vi "Periodic Tasks - working_old.vi"(8 "error in":errorcluster) -> ()   [LabVIEW 2017]
doc: "This VI runs in parallel to other tasks. It can contain as many user-defined periodic loops as you need. These can carry out PID or other sorts of timed response."
uses:
  <vilib>/Analysis/baseanly.llb/Mean (DBL).vi
  <vilib>/Rock Robotics/WPI/Utilities/WPI_GetSetVariantRefNum.vi
  Robot Global Data.vi
  <vilib>/Analysis/NI_AALBase.lvlib
panel:
  out "Avg Y":dbl
  out "Mean":dbl(graph)
  out "Joy Y":dbl(graph)
  out "Current Joy Y Value":dbl
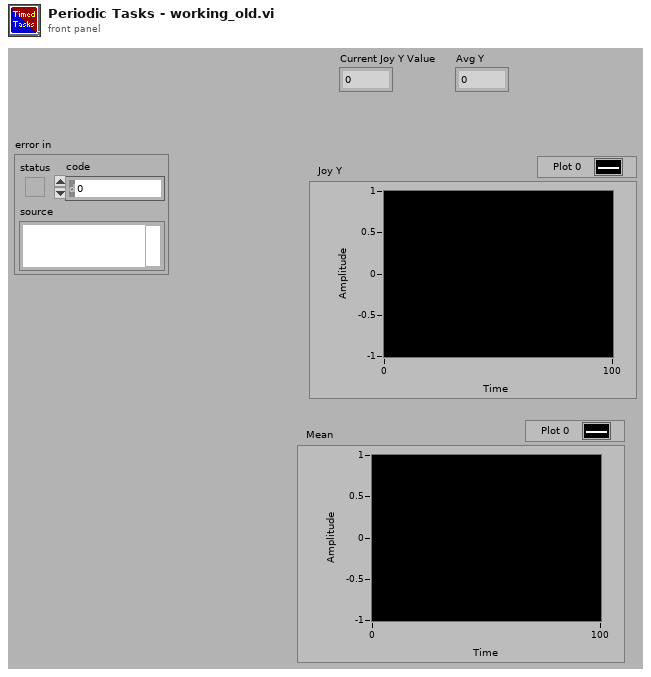
[diagram p1: front panel]
types:
  T1 = typedef "WPI_JoystickDevRef.ctl" = cluster{"Device":T2}
  T2 = typedef "WPI_JoystickDeviceEnum.ctl" = enum16{"USB 0", "USB 1", "USB 2", "USB 3", "USB 4", "USB 5"}
  T3 = typedef "WPI_RobotDriveDevRef.ctl" = cluster{"DevStatus":errorcluster, "Motors[]":T4[], "Square Inputs":bool, "Max Output":dbl}
  T4 = typedef "WPI_MotorControlDeviceRef.ctl" = cluster{"DeviceStatus":errorcluster, "Type":T5, "PWM":cluster{"PWM Channel":T6, "DeadBand":T7}, "CAN":cluster{"Device Number":u8, "SetOutput VI Ref":variant, "GetOutput VI Ref":variant, "Enable VI Ref":variant, "Disable VI Ref":variant, "Data":variant}, "Invert":bool, "DIO PWM":cluster{"PWM \"Enable\" Channel":T6, "DIOChannel":T8, "PWM Rate":dbl}}
  T5 = typedef "WPI_MotorControlType.ctl" = enum16{"PWM", "CAN", "DIO PWM"}
  T6 = typedef "FPGA_DIOPWMChannel.ctl" = enum8{"PWM 0", "PWM 1", "PWM 2", "PWM 3", "PWM 4", "PWM 5", "PWM 6", "PWM 7", "PWM 8", "PWM 9", "PWM MXP 0", "PWM MXP 1", "PWM MXP 2", "PWM MXP 3", "PWM MXP 4", "PWM MXP 5", "PWM MXP 6", "PWM MXP 7", "PWM MXP 8", "PWM MXP 9", "Invalid"}
  T7 = typedef "WPI_PWMDeadband.ctl" = cluster{"Name":string, "maxPositivePwm":i32, "minPositivePwm":i32, "centerPwm":i32, "maxNegativePwm":i32, "minNegativePwm":i32, "angularRange":u16}
  T8 = typedef "FPGA_DIOChannel.ctl" = enum8{"DIO 0", "DIO 1", "DIO 2", "DIO 3", "DIO 4", "DIO 5", "DIO 6", "DIO 7", "DIO 8", "DIO 9", "DIO MXP 0", "DIO MXP 1", "DIO MXP 2", "DIO MXP 3", "DIO MXP 4", "DIO MXP 5", "DIO MXP 6", "DIO MXP 7", "DIO MXP 8", "DIO MXP 9", "DIO MXP 10", "DIO MXP 11", "DIO MXP 12", "DIO MXP 13", "DIO MXP 14", "DIO MXP 15", "SPI Port CS1", "SPI Port CS2", "SPI Port CS3", "SPI Port MISO", "SPI Port MOSI", "Invalid"}
  T9 = cluster{"JoystickDevRef":T1, "RobotDriveDevRef":T3}
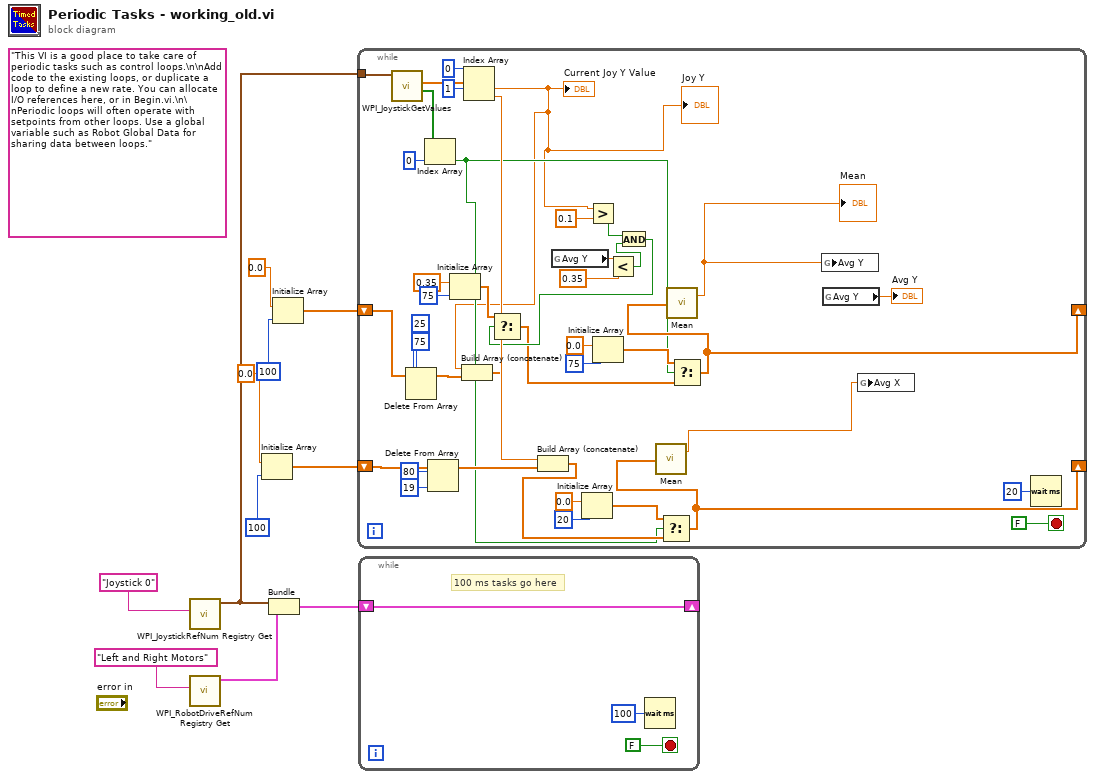
[diagram p0: block diagram]
diagram:
  (unwired) "This VI is a good place to take care of periodic tasks such as control loops.\n\nAdd code to the existing loops, or duplicate a loop to define a new rate. You can allocate I/O references here, or in Begin.vi.\n\nPeriodic loops will often operate with setpoints from other loops. Use a global variable such as Robot Global Data for sharing data between loops."
  n1 = call <vilib>:"WPI_JoystickRefNum Registry Get.vi"("refnum name"="Joystick 0") -> ("JoystickDevRef"=w7:T1)  [unwired: 1 in, 9 out]
  n2 = call <vilib>:"WPI_RobotDriveRefNum Registry Get.vi"("refnum name"="Left and Right Motors") -> ("RobotDriveDevRef"=w9:T3)  [unwired: 1 in, 9 out]
  n3 = Initialize Array(0.0 ("element"), 100 ("dimension size")) -> (w3:dbl[])
  n4 = Bundle("JoystickDevRef"=w7, "RobotDriveDevRef"=w9) -> (w8:T9)  [unwired: 1 out]
  n5 = Initialize Array(0.0 ("element"), 100 ("dimension size")) -> (w4:dbl[])
  n6 = while {
    tunnel: w7 -> [w51]
    shift-right: [w42] -> _
    shift-left: w4 -> [w48]
    shift-right: [w40] -> _
    shift-left: w3 -> [w34]
    stop <- FALSE stop-if-true
    n7 = call <vilib>:"WPI_JoystickGetValues.vi"("JoystickDevRef"=w51) -> ("Buttons"=w47:bool[], "Axes"=w50:dbl[])  [unwired: 6 in, 3 out]
    n8 = Delete From Array(array=w48, length=25, index=75) -> (array with subset deleted=w16:dbl[])  [unwired: 1 out]
    n9 = Index Array(array=w47, index=0) -> (element=w31:bool)
    n10 = Delete From Array(array=w34, length=80, index=19) -> (array with subset deleted=w36:dbl[])  [unwired: 1 out]
    n11 = Initialize Array(0.35 ("element"), 75 ("dimension size")) -> (w26:dbl[])
    n12 = Index Array(array=w50, index #1=1 ("index"), index #2=0 ("index")) -> (element #1=w15:dbl, element #2=w32:dbl)
    "Current Joy Y Value" <- w15
    "Joy Y" <- w15
    n13 = Build Array (concatenate)(w15, w16) -> (w14:dbl[])
    n14 = Build Array (concatenate)(w32, w36) -> (w33:dbl[])
    n15 = global read "Robot Global Data.vi" "Avg Y"() -> (w22:dbl)
    n16 = Initialize Array(0.0 ("element"), 20 ("dimension size")) -> (w39:dbl[])
    n17 = Greater?(x=w15, y=0.1) -> (0:w20:bool)
    n18 = Initialize Array(0.0 ("element"), 75 ("dimension size")) -> (w43:dbl[])
    n19 = Less?(x=w22, y=0.35) -> (x < y?=w19:bool)
    n20 = And(x=w20, y=w19) -> (x .and. y?=w18:bool)
    n21 = Select(t=w26, s=w18, f=w14) -> (s? t:f=w17:dbl[])
    n22 = Select(t=w39, s=w31, f=w33) -> (s? t:f=w40:dbl[])
    n23 = call-poly <vilib>:"Mean.vi"("X"=w40) -> ("mean"=w30:dbl)  [unwired: 1 out]
    n24 = Select(t=w43, s=w31, f=w17) -> (s? t:f=w42:dbl[])
    n25 = call-poly <vilib>:"Mean.vi"("X"=w42) -> ("mean"=w13:dbl)  [unwired: 1 out]
    "Mean" <- w13
    n26 = global write "Robot Global Data.vi" "Avg Y"(w13) -> ()
    n27 = global read "Robot Global Data.vi" "Avg Y"() -> (→"Avg Y":dbl)
    n28 = global write "Robot Global Data.vi" "Avg X"(w30) -> ()
    n29 = Wait (ms)(milliseconds to wait=u32 20) -> ()  [unwired: 1 out]
  }
  n30 = while {
    shift-right: [w54] -> _
    shift-left: w8 -> [w54]
    stop <- FALSE stop-if-true
    # "100 ms tasks go here"
    n31 = Wait (ms)(milliseconds to wait=u32 100) -> ()  [unwired: 1 out]
  }
